vi "Validate_Do.vi"(8 "error in (no error)":errorcluster, 11 "Run System Exec in":refnum<class "Run System Exec.lvclass">) -> (0 "error out":errorcluster, 1 "Valid?":bool, 3 "Run System Exec out":refnum<class "Run System Exec.lvclass">)   [LabVIEW 2020, in "ProjectBuilder.lvlib" / "Run System Exec.lvclass"]
doc: "Override to validate the class.\n\nThe default implementation does nothing but return 'Success?'=True."
uses:
  Run System Exec.lvclass
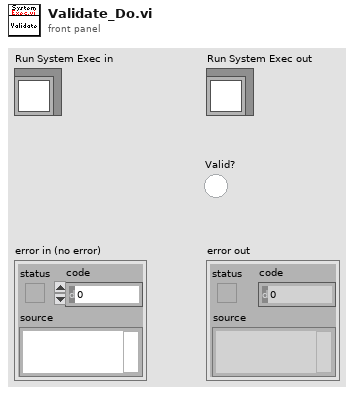
[diagram p1: front panel]
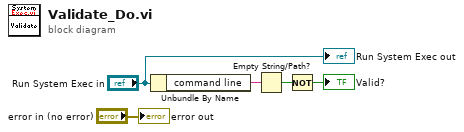
[diagram p0: block diagram]
diagram:
  n1 = Unbundle By Name("Run System Exec in") -> ("command line"=w4:string)
  n2 = Empty String/Path?(string/path=w4) -> (empty?=w3:bool)
  n3 = Not(x=w3) -> (.not. x?=→"Valid?":bool)
  "error out" <- "error in (no error)"
  "Run System Exec out" <- "Run System Exec in"
